vi "Get Consumer Values.vi"(8 "error in":errorcluster, 11 "Cycler Cluster.lvclass in":refnum<class "Cycler Cluster.lvclass">) -> (0 "error out":errorcluster, 1 "Consumer Ch":T2[](array[typedef]), 2 "Consumer Control":T1, 3 "Cycler Cluster.lvclass out":refnum<class "Cycler Cluster.lvclass">)   [LabVIEW 2023, in "Cycler Cluster.lvclass"]
uses:
  Cycler Cluster.lvclass
  Consumer Ch.ctl
  Consumer Control.ctl
  Cycler Cluster.lvclass/Cycler Cluster.ctl
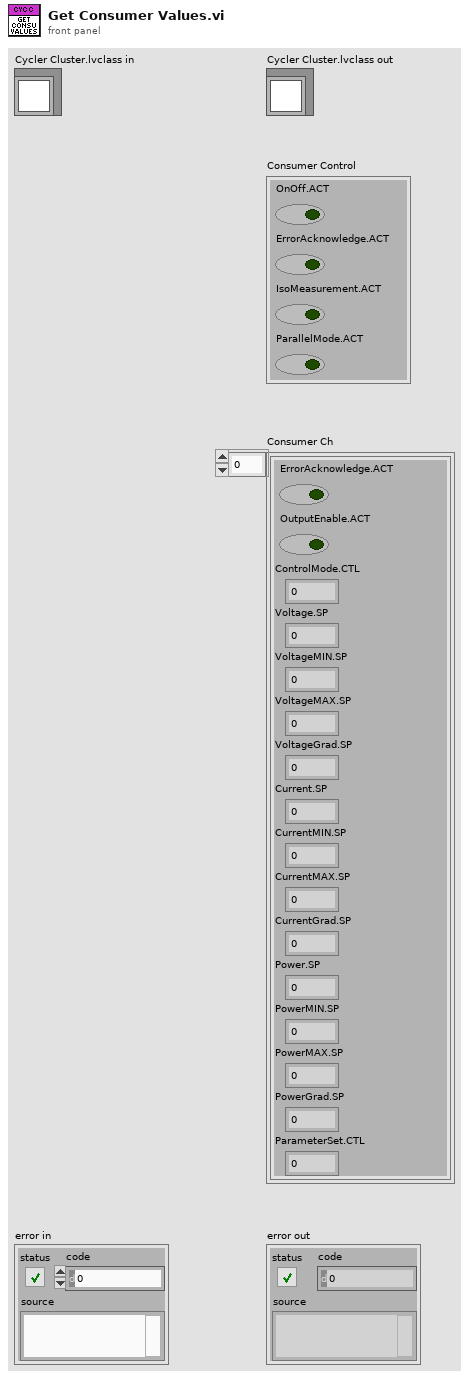
[diagram p1: front panel]
types:
  T1 = typedef "Cycler Cluster.lvclass/Consumer Control.ctl" = cluster{"OnOff.ACT":bool, "ErrorAcknowledge.ACT":bool, "IsoMeasurement.ACT":bool, "ParallelMode.ACT":bool}
  T2 = typedef "Cycler Cluster.lvclass/Consumer Ch.ctl" = cluster{"ErrorAcknowledge.ACT":bool, "OutputEnable.ACT":bool, "ControlMode.CTL":u16, "Voltage.SP":dbl, "VoltageMIN.SP":dbl, "VoltageMAX.SP":dbl, "VoltageGrad.SP":dbl, "Current.SP":dbl, "CurrentMIN.SP":dbl, "CurrentMAX.SP":dbl, "CurrentGrad.SP":dbl, "Power.SP":dbl, "PowerMIN.SP":dbl, "PowerMAX.SP":dbl, "PowerGrad.SP":dbl, "ParameterSet.CTL":i32}
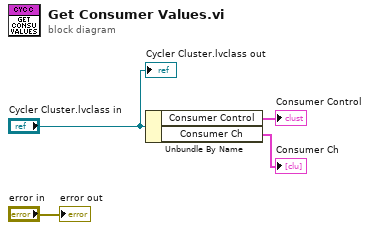
[diagram p0: block diagram]
diagram:
  n1 = Unbundle By Name("Cycler Cluster.lvclass in") -> ("Consumer Control"=→"Consumer Control":T1, "Consumer Ch"=→"Consumer Ch":T2[])
  "error out" <- "error in"
  "Cycler Cluster.lvclass out" <- "Cycler Cluster.lvclass in"
